vi "3CH.vi"() -> ()   [LabVIEW 2024]
uses:
  <vilib>/Instr/_visa.llb/VISA Configure Serial Port (Instr).vi
  <vilib>/Utility/file.llb/Write Delimited Spreadsheet (DBL).vi
panel:
  in  "stop 2":bool
  out "element":sgl[](array[numeric])
  in  "file path  2":path=path "C:/temp/test1.txt"
  out "error out 2":errorcluster
  in  "VISA resource name":refnum<visa-resource-name>="COM8"
  out "Waveform Chart":sgl[][](graph)
  out "dt (ms)":u32
  out "freq (hz)":dbl
  out "Number of Bytes at Serial Port":u32
  out "byte read count":u32
  in  "stop":bool
  out "read buffer":string
  # "NB: record data until STOP is pressed"
  # "Add a file name!"
  # "Select!"
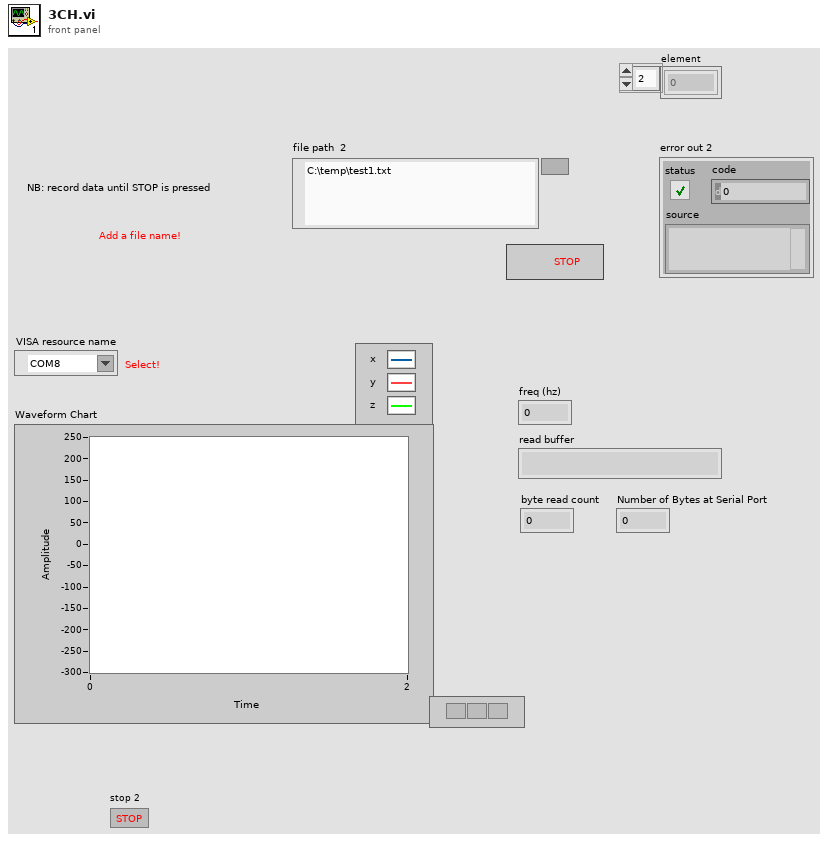
[diagram p1: front panel]
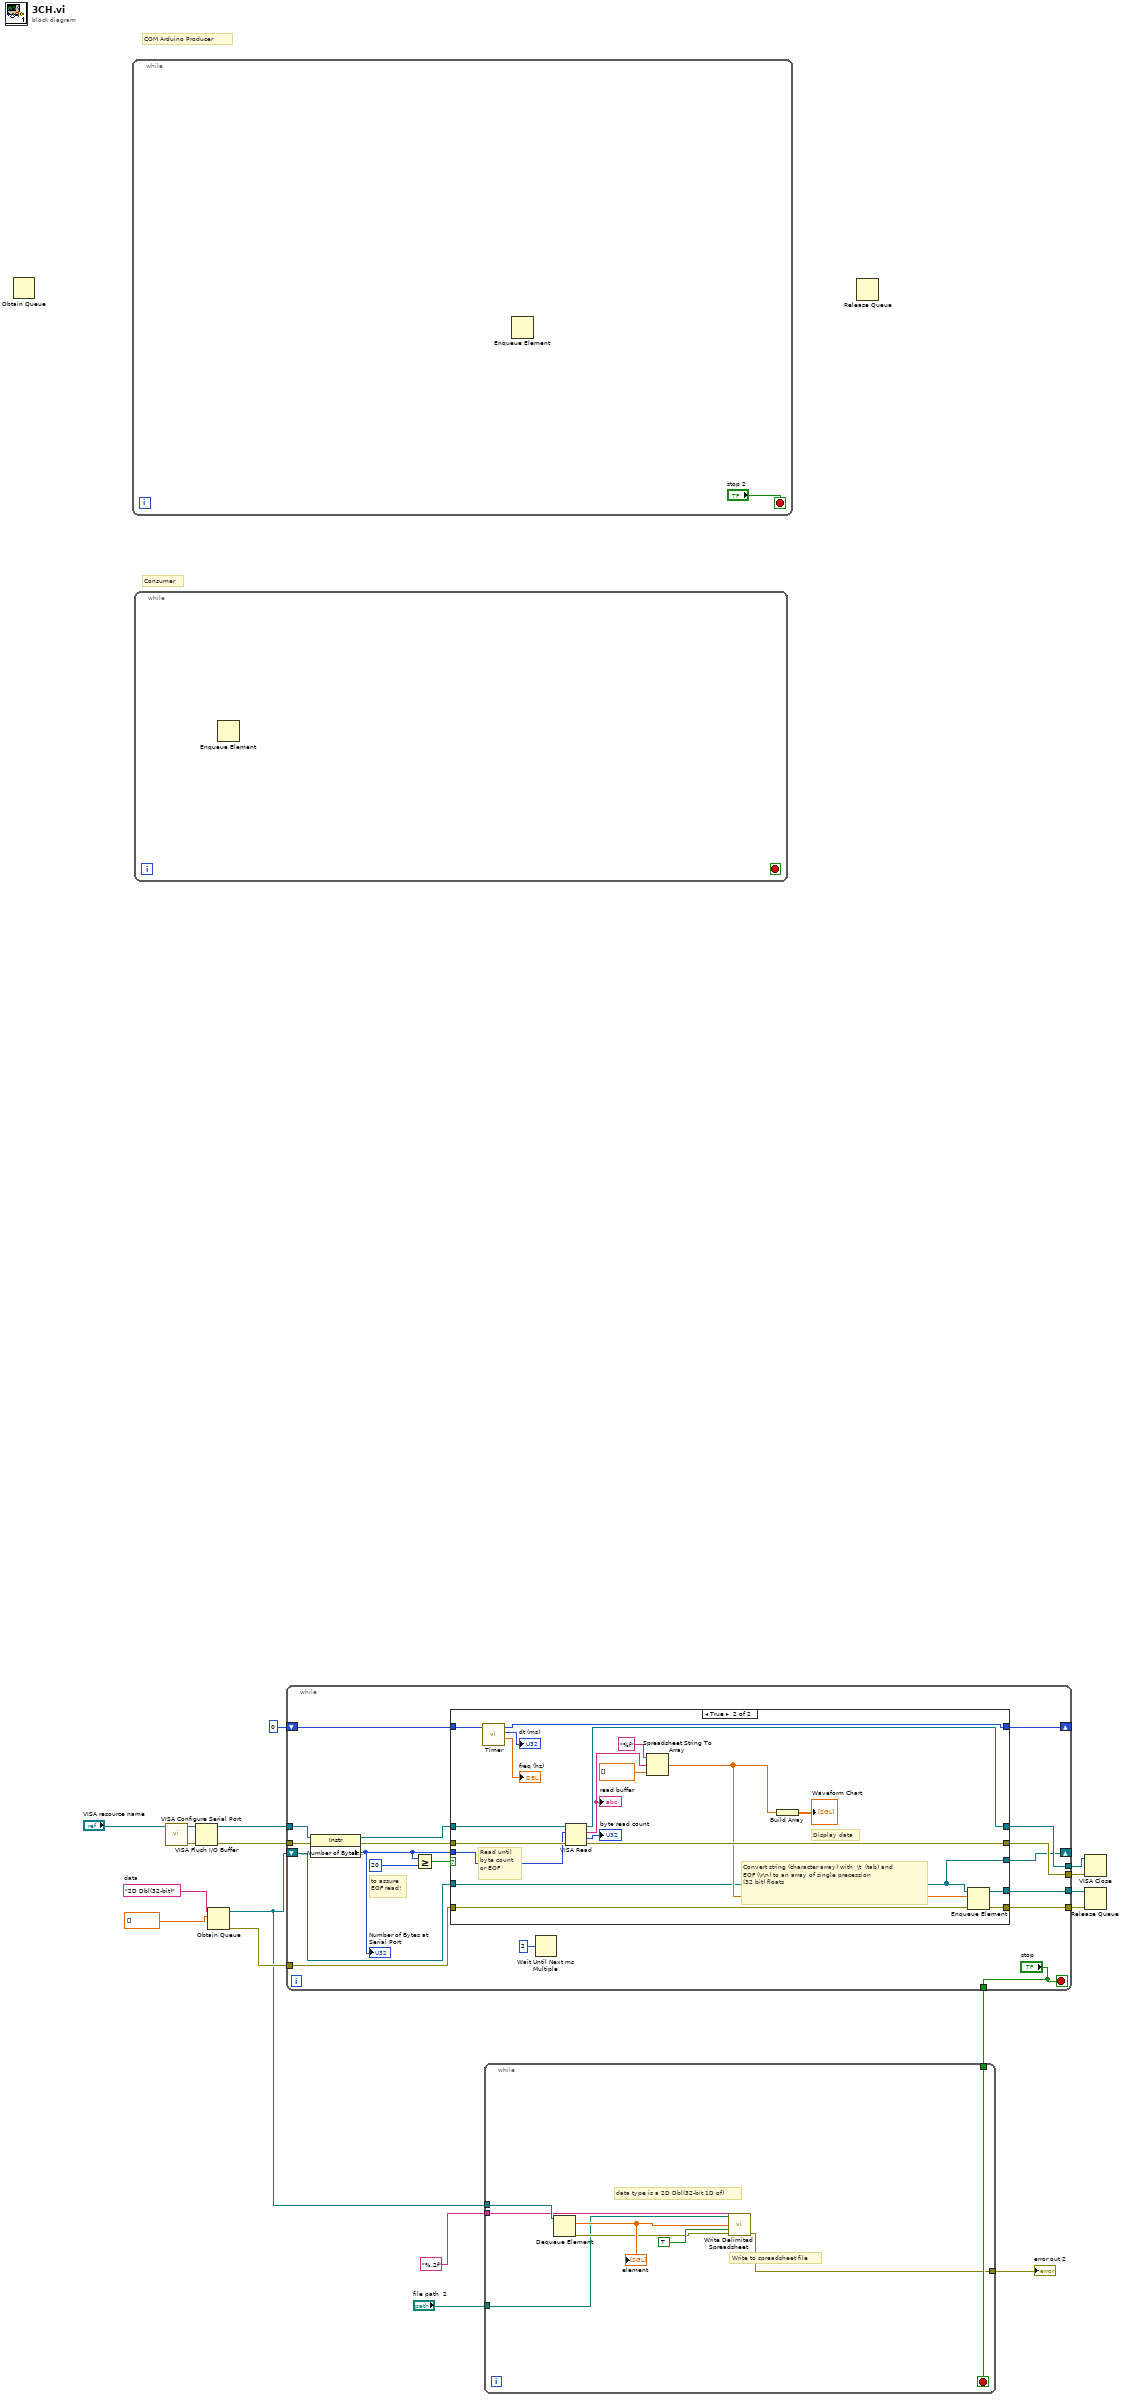
[diagram p0: block diagram]
diagram:
  w6 = "2D Dbl(32-bit)"  # data
  # "Consumer"
  # "COM Arduino Producer"
  n1 = Obtain Queue() -> ()  [unwired: 5 in, 3 out]
  n2 = while {
    stop <- "stop 2" stop-if-true
    n3 = Enqueue Element() -> ()  [unwired: 4 in, 3 out]
  }
  n4 = while {
    stop <- _ stop-if-true
    n5 = Enqueue Element() -> ()  [unwired: 4 in, 3 out]
  }
  n6 = call-poly "VISA Configure Serial Port"("VISA resource name"="VISA resource name") -> ("VISA resource name out"=w15:refnum<visa-resource-name>, "error out"=w14:errorcluster)  [unwired: 13 in]
  n7 = VISA Flush I/O Buffer(VISA resource name=w15, error in (no error)=w14) -> (VISA resource name out=w13:refnum<visa-resource-name>, error out=w12:errorcluster)  [unwired: 1 in]
  n8 = Obtain Queue(name (unnamed)=w6, element data type=sgl[] [] ("array type (2D Dbl)")) -> (queue out=w5:refnum<queue>, error out=w10:errorcluster)  [unwired: 3 in, 1 out]
  n9 = while {
    tunnel: w13 -> [w37]
    tunnel: w12 -> [w36]
    tunnel: [w33] -> w17
    tunnel: [w32] -> w16
    shift-right: [w26] -> _
    shift-left: u32 0 -> [w27]
    shift-right: [w21] -> _
    shift-left: w5 -> [w25]
    tunnel: w10 -> [w24]
    tunnel: [w23] -> w9
    tunnel: [w22] -> w8
    tunnel: ["stop"] -> w4
    stop <- "stop" stop-if-true
    # "to assure\nEOF read!"
    n10 = property class="Instr"(reference=w37, error in=w36) -> (reference out=w34:refnum<visa-resource-name>, error out=w35:errorcluster, "Serial Settings:Number of Bytes at Serial Port"=w29:u32)
    "Number of Bytes at Serial Port" <- w29
    n11 = Greater Or Equal?(x=w29, y=u32 20) -> (x >= y?=w30:bool)
    n12 = case shown="True" w30 {
      tunnel: w35 -> [w41 w61]
      tunnel: w34 -> [w42 w60]
      tunnel: w29 -> [_ w59]
      tunnel: [w42 w58] -> w33
      tunnel: [w41 w57] -> w32
      tunnel: w27 -> [w40 w55]
      tunnel: [w40 w54] -> w26
      tunnel: w25 -> [w38 w43]
      tunnel: w24 -> [w39 w47]
      tunnel: [w38 w46] -> w23
      tunnel: [w39 w45] -> w22
      tunnel: [w38 w43] -> w21
      frame False {
      }
      frame True {
        # "Display data"
        # "Convert string (character array) with  \\t  (tab) and \nEOF (\\r\\n) to an array of single precession \n(32 bit) floats"
        # "Read until\nbyte count\nor EOF"
        n13 = call "Timer.vi"("Previous_ms"=w55) -> ("freq (hz)"=→"freq (hz)":dbl, "dt (ms)"=→"dt (ms)":u32, "Next_ms"=w54:u32)  [unwired: 8 in]
        n14 = VISA Read(VISA resource name=w60, byte count=w59, error in (no error)=w61) -> (VISA resource name out=w58:refnum<visa-resource-name>, read buffer=w49:string, return count=→"byte read count":u32, error out=w57:errorcluster)
        "read buffer" <- w49
        n15 = Spreadsheet String To Array(format string="%f", spreadsheet string=w49, array type (2D Dbl)=sgl[] []) -> (array=w44:sgl[])  [unwired: 1 in]
        n16 = Build Array(w44) -> (→"Waveform Chart":sgl[][])
        n17 = Enqueue Element(queue=w43, element=w44, error in (no error)=w47) -> (queue out=w46:refnum<queue>, error out=w45:errorcluster)  [unwired: 1 in, 1 out]
      }
    }
    n18 = Wait Until Next ms Multiple(millisecond multiple=u32 2) -> ()  [unwired: 1 out]
  }
  n19 = while {
    tunnel: w5 -> [w68]
    tunnel: w4 -> [w66]
    tunnel: "file path  2" -> [w64]
    tunnel: "%.2f" ("format (%.3f)") -> [w63]
    tunnel: [w62] -> w1
    stop <- w66 stop-if-true
    # "data type is a 2D Dbl(32-bit 1D of)"
    # "Write to spreadsheet file"
    n20 = Dequeue Element(queue=w68) -> (element=w67:sgl[], error out=w65:errorcluster)  [unwired: 2 in, 2 out]
    "element" <- w67
    n21 = call-poly <vilib>:"Write Delimited Spreadsheet.vi"("file path (dialog if empty)"=w64, "format (%.3f)"=w63, "1D data"=w67, "append to file? (new file:F)"=TRUE, "error in (no error)"=w65) -> ("error out"=w62:errorcluster)  [unwired: 9 in, 1 out]
  }
  "error out 2" <- w1
  n22 = Release Queue() -> ()  [unwired: 3 in, 3 out]
  n23 = VISA Close(VISA resource name=w17, error in (no error)=w16) -> ()  [unwired: 1 out]
  n24 = Release Queue(queue=w9, error in (no error)=w8) -> ()  [unwired: 1 in, 3 out]
